vi "function4.vi"(1 "Input":dbl) -> (0 "Output":dbl)   [LabVIEW 2012]
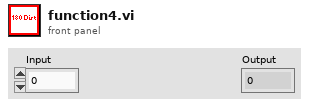
[diagram p1: front panel]
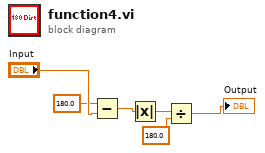
[diagram p0: block diagram]
diagram:
  n1 = Subtract(x=180.0, y="Input") -> (x-y=w4:dbl)
  n2 = Absolute Value(x=w4) -> (abs(x)=w3:dbl)
  n3 = Divide(x=w3, y=180.0) -> (x/y=→"Output":dbl)
